vi "projectileCalc.vi"() -> ()   [LabVIEW 2020]
panel:
  out "lauch angle":dbl
  in  "velocity":dbl
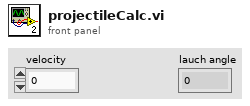
[diagram p1: front panel]
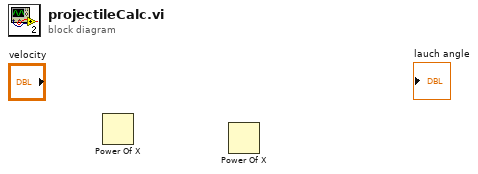
[diagram p0: block diagram]
diagram:
  n1 = Power Of X() -> ()  [unwired: 2 in, 1 out]
  n2 = Power Of X() -> ()  [unwired: 2 in, 1 out]
